vi "To String Tree Data.vi"(10 "String":string) -> (3 "String Tree Data":refnum<class "String.lvclass">)   [LabVIEW 2017, in "Tree API.lvlib" / "String.lvclass"]
doc: "Convert a String value to Tree Data type."
uses:
  String.lvclass
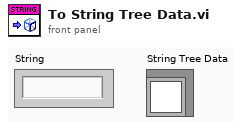
[diagram p1: front panel]
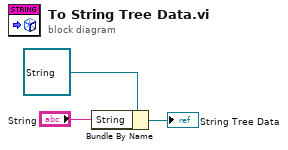
[diagram p0: block diagram]
diagram:
  n1 = Bundle By Name(cluster=refnum<class "String.lvclass"> refnum ("String in"), "String"="String") -> (→"String Tree Data":refnum<class "String.lvclass">)
